vi "Check Is Test Case.vi"(11 "reference in":refnum<vi>) -> (2 "Is Test Case?":bool, 3 "reference out":refnum<vi>)   [LabVIEW 2020, in "Icon Decorator.lvlib" / "Icon Decorator.lvclass"]
uses:
  Icon Decorator.lvclass
  LUnit Test Case.lvclass
  Icon Decorator.lvclass/Icon Decorator.ctl
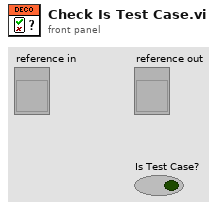
[diagram p1: front panel]
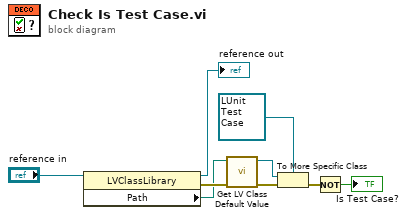
[diagram p0: block diagram]
diagram:
  n1 = property class="LVClassLibrary"(reference="reference in") -> (reference out=→"reference out":refnum<vi>, error out=w5:errorcluster, "Path"=w4:path)  [unwired: 1 in]
  n2 = call <vilib>:"Get LV Class Default Value.vi"("error in (no error)"=w5, "class path"=w4) -> ("error out"=w7:errorcluster, "object"=w6:refnum<class>)  [unwired: 8 in]
  n3 = To More Specific Class(target class=refnum<class "LUnit Test Case.lvclass"> refnum ("LUnit Test Case V2.lvclass"), reference=w6, error in=w7) -> (error out=w3:errorcluster)  [unwired: 1 out]
  n4 = Not(x=w3) -> (.not. x?=→"Is Test Case?":bool)
